vi "Write SysHandle.vi"(8 "error in (no error)":errorcluster, 10 "SysHandle":refnum<k21>, 11 "NiPxi6682 in":refnum<class "NiPxi6682.lvclass">) -> (0 "error out":errorcluster, 3 "NiPxi6682 out":refnum<class "NiPxi6682.lvclass">)   [LabVIEW 2014, in "SyncPlugins.lvlib" / "NiPxi6682.lvclass"]
uses:
  NiPxi6682.lvclass
  NiPxi6682.lvclass/NiPxi6682.ctl
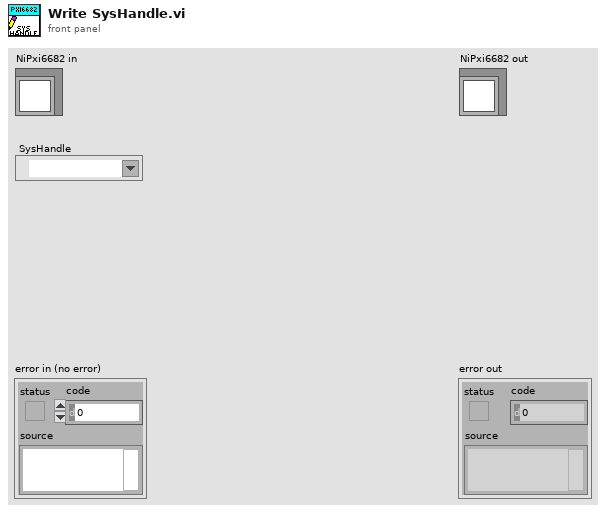
[diagram p1: front panel]
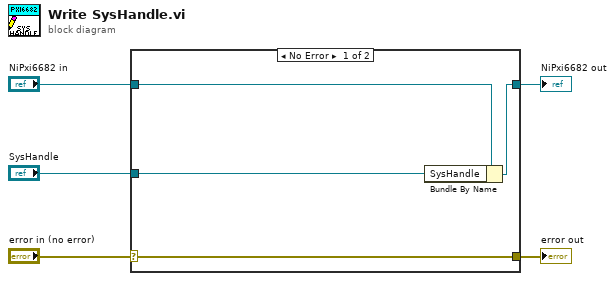
[diagram p0: block diagram]
diagram:
  n1 = case shown="No Error" "error in (no error)" {
    selector: "error in (no error)" -> [w9 w10]
    tunnel: [w9 w10] -> w4
    tunnel: [w7 w11] -> w2
    tunnel: "NiPxi6682 in" -> [w8 w11]
    tunnel: "SysHandle" -> [w6 _]
    frame No Error {
      n2 = Bundle By Name(cluster=w8, "SysHandle"=w6) -> (w7:refnum<class "NiPxi6682.lvclass">)
    }
    frame Error {
    }
  }
  "error out" <- w4
  "NiPxi6682 out" <- w2
